vi "create input request.vi"(11 "input request":T1[](array[typedef])) -> (3 "request w/o header":u32[](array[numeric]))   [LabVIEW 2013, in "dynamic profibus.lvlib"]
uses:
  dynamic profibus.lvlib
  input request.ctl
  profibus master action.ctl
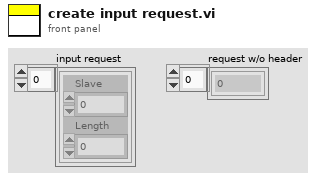
[diagram p1: front panel]
types:
  T1 = typedef "dynamic profibus.lvlib/input request.ctl" = cluster{"Slave":u8, "Length":u8}
  T2 = typedef "profibus master action.ctl" = enum8{"set output", "transfer complete", "configure reads", "configure diagnostics"}
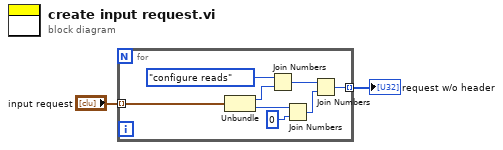
[diagram p0: block diagram]
diagram:
  n1 = for {
    tunnel: "input request" -> [w10] mode=indexing
    tunnel: [w3] -> w2 mode=indexing
    n2 = Unbundle(w10) -> ("Slave"=w6:u8, "Length"=w5:u8)
    n3 = Join Numbers(hi=profibus_master_action."configure reads" ("action"), lo=w6) -> ((hi.lo)=w9:u16)
    n4 = Join Numbers(hi=w5, lo=u8 0) -> ((hi.lo)=w8:u16)
    n5 = Join Numbers(hi=w9, lo=w8) -> ((hi.lo)=w3:u32)
  }
  "request w/o header" <- w2
